vi "Speed to Samples.vi"(1 "Distancias generales (m)":dbl[](array[numeric]), 2 "Loop Rate (Hz)":dbl, 3 "Velocidad de eje(m/s)":dbl[](array[numeric])) -> (0 "Longitud de ventana (puntos)":dbl[](array[numeric]))   [LabVIEW 2015]
doc: "Se calculan los puntos de las ventana de cada rueda, en función de la velocidad del eje y de la distancia de configuración en metros de la ventana"
panel:
  in  "Tamaño de la ventana":dbl=2.64
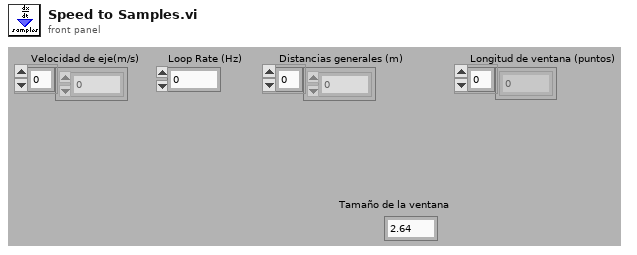
[diagram p1: front panel]
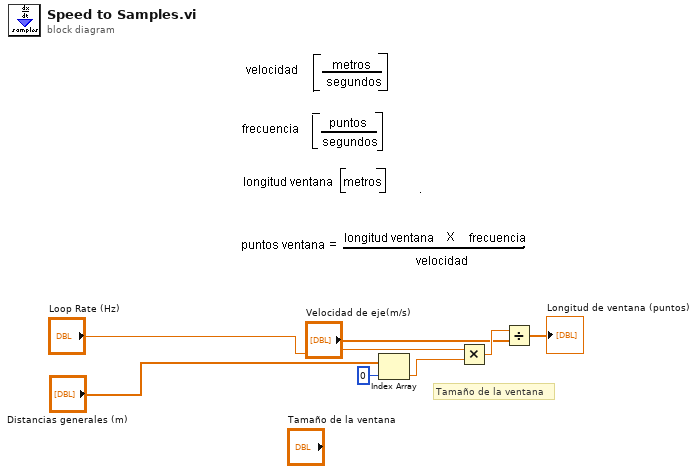
[diagram p0: block diagram]
diagram:
  # "Tamaño de la ventana"
  n1 = Index Array(array="Distancias generales (m)", index=0) -> (element=w1:dbl)
  n2 = Multiply(x="Loop Rate (Hz)", y=w1) -> (x*y=w6:dbl)
  n3 = Divide(x=w6, y="Velocidad de eje(m/s)") -> (x/y=→"Longitud de ventana (puntos)":dbl[])
